vi "cook.vi"(8 "error in (no error)":errorcluster, 11 "Appliance in":refnum<class "Appliance.lvclass">) -> (0 "error out":errorcluster, 3 "Appliance out":refnum<class "Appliance.lvclass">)   [LabVIEW 2011, in "Appliance.lvclass"]
uses:
  Appliance.lvclass
  Appliance.lvclass/Appliance.ctl
  CookBehavior/CookBehavior.lvclass
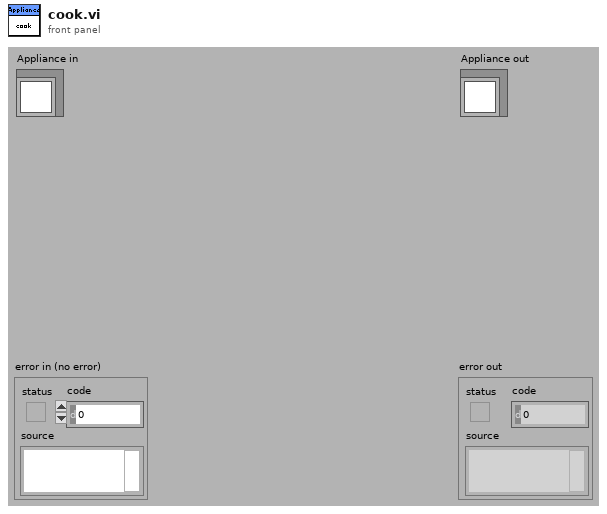
[diagram p1: front panel]
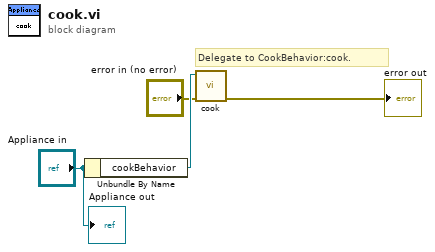
[diagram p0: block diagram]
diagram:
  # "Delegate to CookBehavior:cook."
  n1 = Unbundle By Name("Appliance in") -> ("cookBehavior"=w2:refnum<class "CookBehavior.lvclass">)
  n2 = call-dynamic "cook.vi"("error in (no error)"="error in (no error)", "CookBehavior in"=w2) -> ("error out"=→"error out":errorcluster)  [unwired: 8 in, 1 out]
  "Appliance out" <- "Appliance in"
